vi "Send to Volt Meter.vi"(0 "Address":string="24", 1 "Data":string) -> ()   [LabVIEW 2012]
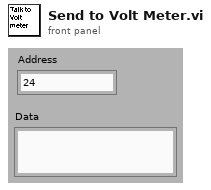
[diagram p1: front panel]
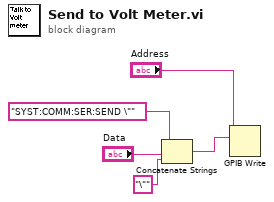
[diagram p0: block diagram]
diagram:
  n1 = Concatenate Strings("SYST:COMM:SER:SEND \"" ("string"), "Data", "\"" ("string")) -> (w5:string)
  n2 = GPIB Write(0:"Address", 1:w5) -> ()  [unwired: 3 in, 2 out]
